vi "Initialize Default.vi"(8 "error in (no error)":errorcluster, 11 "DSF Buffer Converter Transfer Configuration in":refnum<class "Default Buffer Converter Transfer Configuration.lvclass">) -> (0 "error out":errorcluster, 3 "DSF Buffer Converter Transfer Configuration out":refnum<class "Default Buffer Converter Transfer Configuration.lvclass">)   [LabVIEW 2021, in "DSF Core.lvlib" / "Default Buffer Converter Transfer Configuration.lvclass"]
uses:
  Default Buffer Converter Transfer Configuration.lvclass
  Typedefs/DSF Byte Order.ctl
  Default Buffer Converter Transfer Configuration.lvclass/Default Buffer Converter Transfer Configuration.ctl
  DSF Core.lvlib
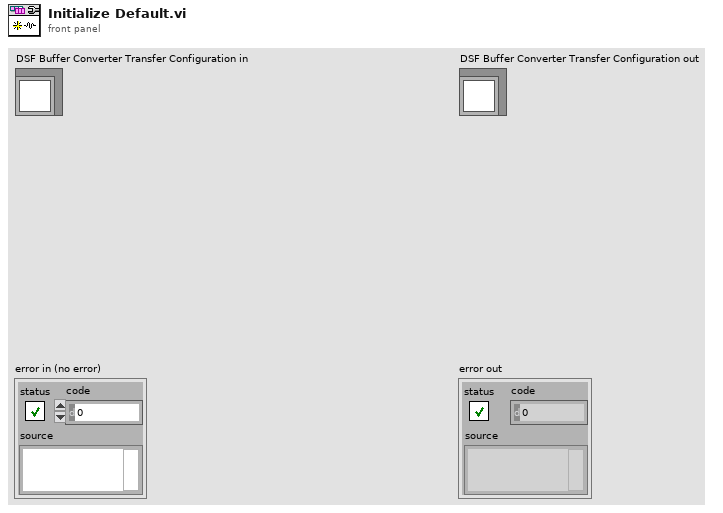
[diagram p1: front panel]
types:
  T1 = typedef "DSF Core.lvlib/DSF Byte Order.ctl" = enum8{"big-endian", "little-endian"}
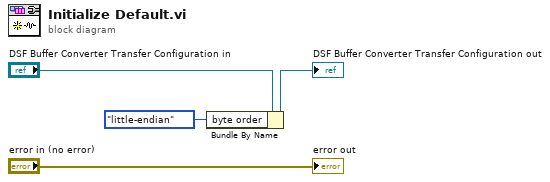
[diagram p0: block diagram]
diagram:
  n1 = Bundle By Name(cluster="DSF Buffer Converter Transfer Configuration in", "byte order"=DSF_Byte_Order."little-endian" ("configuration.byte order")) -> (→"DSF Buffer Converter Transfer Configuration out":refnum<class "Default Buffer Converter Transfer Configuration.lvclass">)
  "error out" <- "error in (no error)"
